vi "Get_KPRO_data_from_file 2016.vi"(11 "Output File KPRO Test":path=path "c:/KPRO_001.txt") -> (0 "Last_height_of_box":dbl format="%.2f", 1 "Last_depth_to_water":dbl format="%.2f", 2 "Last_depth":dbl format="%.2f", 3 "Output_array":sgl[][](array[numeric]) format="%.2f")   [LabVIEW 2016]
uses:
  <vilib>/Utility/file.llb/Read Delimited Spreadsheet (DBL).vi
panel:
  out "report_header_length":i32
  out "Report_header_string":string
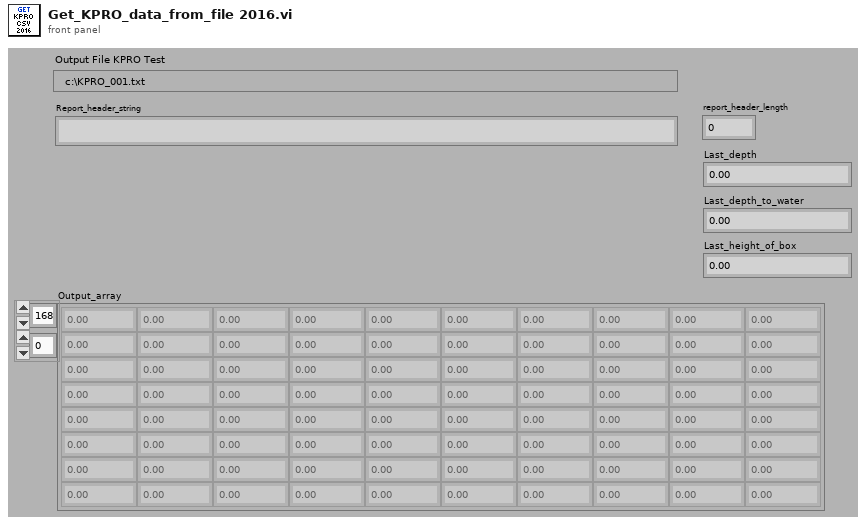
[diagram p1: front panel]
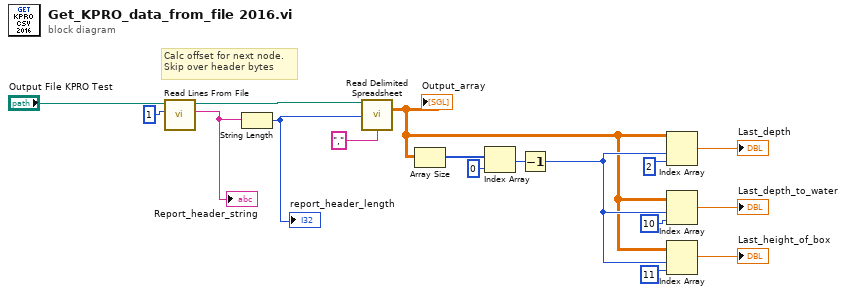
[diagram p0: block diagram]
diagram:
  # "Calc offset for next node.\nSkip over header bytes"
  n1 = call <vilib>:"Read Lines From File.vi"("file path (dialog if empty)"="Output File KPRO Test", "number of lines (all:-1)"=1) -> ("new file path (Not A Path if cancelled)"=w13:path, "line string"=w15:string)  [unwired: 4 in, 2 out]
  "Report_header_string" <- w15
  n2 = String Length(string=w15) -> (length=w17:i32)
  "report_header_length" <- w17
  n3 = call-poly <vilib>:"Read Delimited Spreadsheet.vi"("file path (dialog if empty)"=w13, "start of read offset (chars.:0)"=w17, "delimiter (\\t)"="," ("delimiter (\\t)")) -> ("all rows"=w4:dbl[][])  [unwired: 7 in, 5 out]
  "Output_array" <- w4
  n4 = Array Size(array=w4) -> (size(s)=w11:i32[])
  n5 = Index Array(array=w11, index=0) -> (element=w9:i32)
  n6 = Decrement(x=w9) -> (x-1=w7:i32)
  n7 = Index Array(array=w4, index (row)=w7, index (col)=2 ("index")) -> (element=→"Last_depth":dbl)
  n8 = Index Array(array=w4, index (row)=w7, index (col)=10 ("disabled index (col)")) -> (element=→"Last_depth_to_water":dbl)
  n9 = Index Array(array=w4, index (row)=w7, index (col)=11 ("index")) -> (element=→"Last_height_of_box":dbl)
